vi "Odometry Reset.vi"(8 "error in (no error)":errorcluster, 11 "Reset? (T)":bool=TRUE) -> (0 "error out":errorcluster)   [LabVIEW 2017]
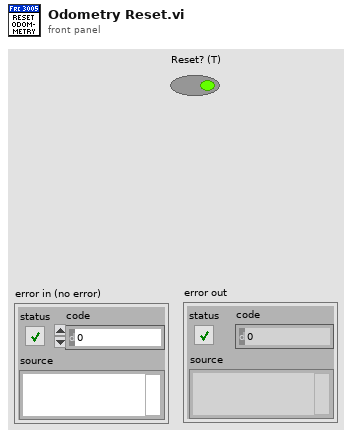
[diagram p1: front panel]
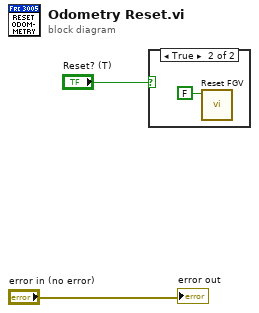
[diagram p0: block diagram]
diagram:
  n1 = case shown="True" "Reset? (T)" {
    frame False {
    }
    frame True {
      n2 = call "Reset FGV.vi"("Get? (T)"=FALSE) -> ()  [unwired: 10 in, 1 out]
    }
  }
  "error out" <- "error in (no error)"
